vi "Read CSV (SubVI).vi"() -> (3 "Data Out":T1[](array[typedef]))   [LabVIEW 2019]
uses:
  Exercise 12/CLD 12 Data Cluster.ctl
  Exercise 12/CLD 12 Sequencer Enum.ctl
  <vilib>/Utility/file.llb/Read Delimited Spreadsheet (string).vi
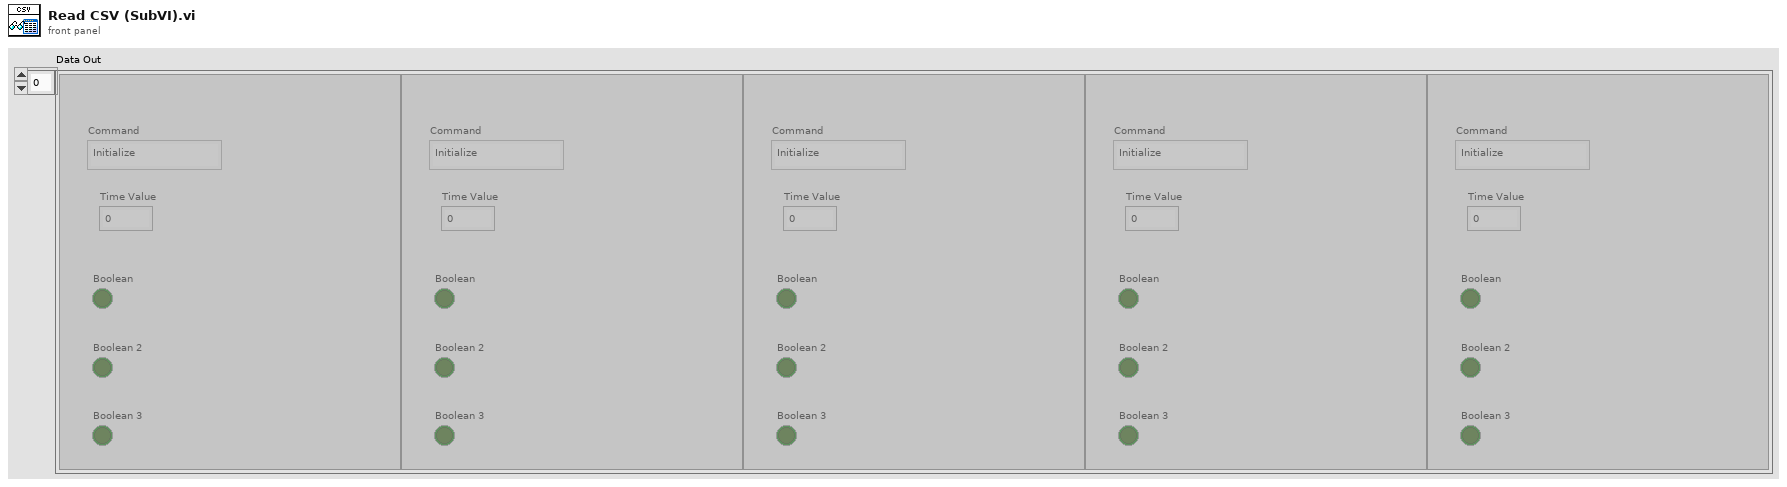
[diagram p1: front panel]
types:
  T1 = typedef "CLD 12 Data Cluster.ctl" = cluster{"Command":T2, "Time Value":dbl, "Boolean":bool, "Boolean 2":bool, "Boolean 3":bool}
  T2 = typedef "CLD 12 Sequencer Enum.ctl" = enum16{"Initialize", "SetTime", "RunState1", "Runstate2", "Idle", "Start"}
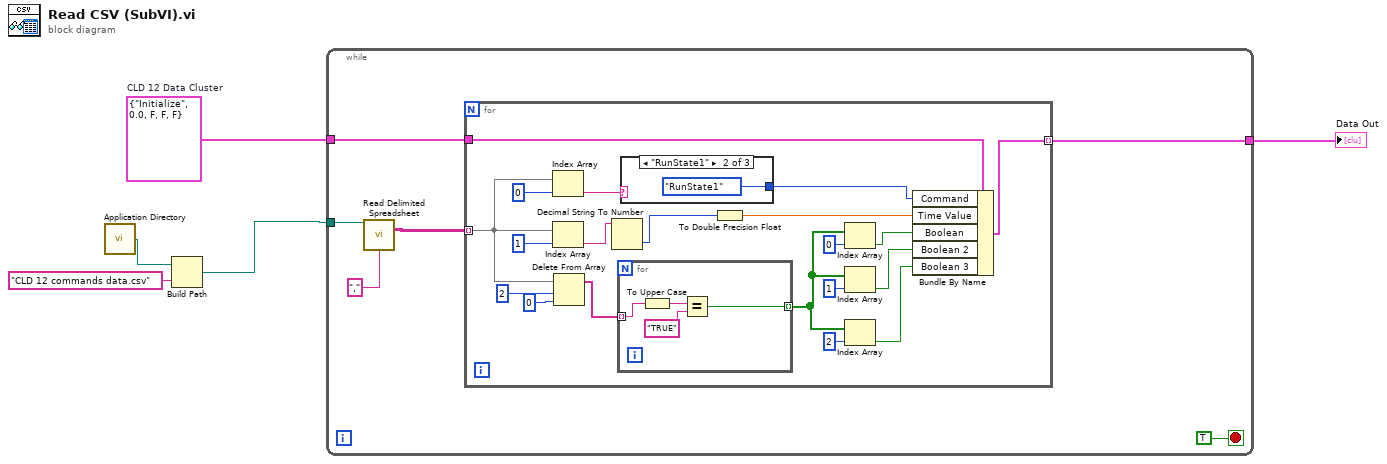
[diagram p0: block diagram]
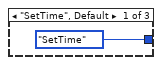
[diagram p2: hidden frame]
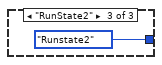
[diagram p3: hidden frame]
diagram:
  w2 = T1 {"Command"=enum."Initialize", "Time Value"=0.0, "Boolean"=FALSE, "Boolean 2"=FALSE, "Boolean 3"=FALSE}  # CLD 12 Data Cluster
  n1 = call <vilib>:"Application Directory.vi"() -> ("Application Directory"=w5:path)
  n2 = Build Path(base path=w5, name or relative path="CLD 12 commands data.csv") -> (appended path=w3:path)
  n3 = while {
    tunnel: w3 -> [w10]
    tunnel: w2 -> [w7]
    tunnel: [w6] -> w1
    stop <- TRUE stop-if-true
    n4 = call-poly <vilib>:"Read Delimited Spreadsheet.vi"("file path (dialog if empty)"=w10, "delimiter (\\t)"="," ("delimiter (\\t)")) -> ("all rows"=w9:string[][])  [unwired: 8 in, 5 out]
    n5 = for {
      tunnel: w9 -> [w23] mode=indexing
      tunnel: w7 -> [w30]
      tunnel: [w20] -> w6 mode=indexing
      n6 = Index Array(array=w23, index=0) -> (element=w29:string)
      n7 = Index Array(array=w23, index=1) -> (element=w26:string)
      n8 = Delete From Array(array=w23, length=2, index=0) -> (array with subset deleted=w19:string[])  [unwired: 1 out]
      n9 = Decimal String To Number(string=w26) -> (number=w25:i32)  [unwired: 2 in, 1 out]
      n10 = for {
        tunnel: w19 -> [w35] mode=indexing
        tunnel: [w32] -> w18 mode=indexing
        n11 = To Upper Case(1:w35) -> (0:w34:string)
        n12 = Equal?(x=w34, y="TRUE") -> (x = y?=w32:bool)
      }
      n13 = case shown="\"RunState1\"" w29 {
        tunnel: [CLD_12_Sequencer_Enum."SetTime" ("CLD 12 Sequencer Control") CLD_12_Sequencer_Enum."RunState1" ("CLD 12 Sequencer Control") CLD_12_Sequencer_Enum."Runstate2" ("CLD 12 Sequencer Control")] -> w28
        frame "SetTime", Default {
        }
        frame "RunState1" {
        }
        frame "RunState2" {
        }
      }
      n14 = To Double Precision Float(number=w25) -> (double precision float=w24:dbl)
      n15 = Index Array(array=w18, index=0) -> (element=w14:bool)
      n16 = Index Array(array=w18, index=1) -> (element=w13:bool)
      n17 = Index Array(array=w18, index=2) -> (element=w12:bool)
      n18 = Bundle By Name(cluster=w30, "Command"=w28, "Time Value"=w24, "Boolean"=w14, "Boolean 2"=w13, "Boolean 3"=w12) -> (w20:T1)
    }
  }
  "Data Out" <- w1
